vi "Find Available Queue.vi"() -> (3 "String":string)   [LabVIEW 2020]
uses:
  <userlib>/RxnRover/DynamicReentrant/src/Type Defs/Message.ctl
  <userlib>/RxnRover/DynamicReentrant/Dynamic Reentrant.lvlib
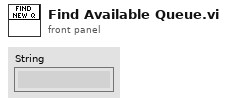
[diagram p1: front panel]
types:
  T1 = typedef "Dynamic Reentrant.lvlib/Message.ctl" = cluster{"Source":string, "Destination":string, "Time Stamp":timestamp, "Command":string, "Data":variant}
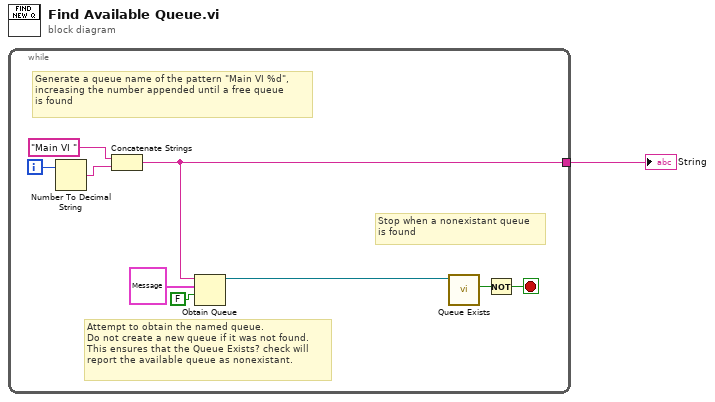
[diagram p0: block diagram]
diagram:
  n1 = while {
    tunnel: [w3] -> w1
    i -> [w6]
    stop <- w9 stop-if-true
    # "Generate a queue name of the pattern \"Main VI %d\",\nincreasing the number appended until a free queue\nis found"
    # "Attempt to obtain the named queue.\nDo not create a new queue if it was not found.\nThis ensures that the Queue Exists? check will\nreport the available queue as nonexistant."
    # "Stop when a nonexistant queue\nis found"
    n2 = Number To Decimal String(number=w6) -> (decimal integer string=w4:string)  [unwired: 1 in]
    n3 = Concatenate Strings("Main VI ", w4) -> (w3:string)
    n4 = Obtain Queue(name (unnamed)=w3, element data type=T1 {"Source"="", "Destination"="", "Time Stamp"=timestamp(0 s since 1904-01-01), "Command"="", "Data"=variant} ("Message"), create if not found? (T)=FALSE) -> (queue out=w8:refnum<queue>)  [unwired: 2 in, 2 out]
    n5 = call <userlib>:"Queue Exists.vi"("Remote VI Queue in"=w8) -> ("Queue Exists"=w10:bool)  [unwired: 9 in, 1 out]
    n6 = Not(x=w10) -> (.not. x?=w9:bool)
  }
  "String" <- w1
